vi "Find tab index.vi"(8 "error in (no error)":errorcluster, 11 "Save Image in":refnum<class "Save Image.lvclass">) -> (0 "error out":errorcluster, 1 "column":i32, 2 "row":i32, 3 "Save Image out":refnum<class "Save Image.lvclass">)   [LabVIEW 2018, in "Save Image.lvclass"]
uses:
  Save Image.lvclass
  Save Image.lvclass/Save Image.ctl
  Simulated_Header/Simulated_Header.lvclass
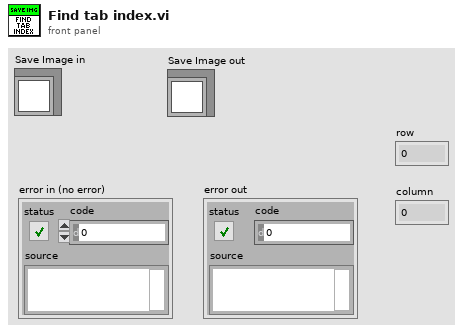
[diagram p1: front panel]
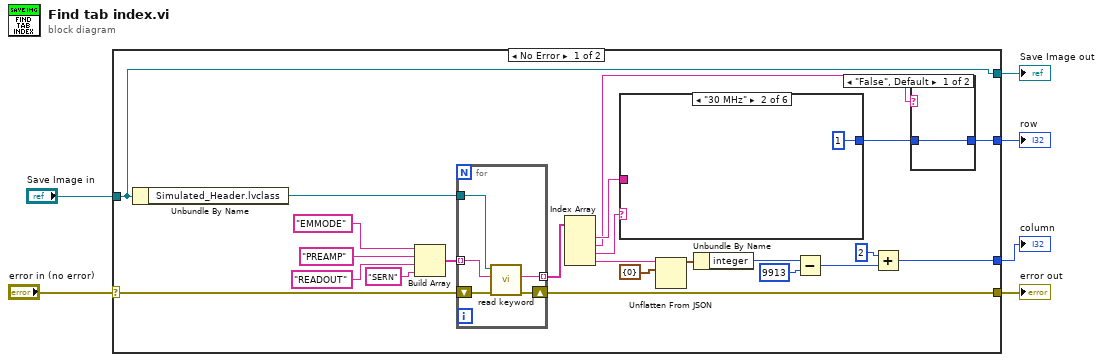
[diagram p0: block diagram]
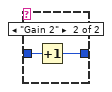
[diagram p2: hidden frame]
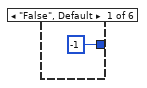
[diagram p3: hidden frame]
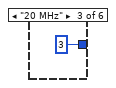
[diagram p4: hidden frame]
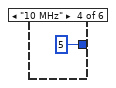
[diagram p5: hidden frame]
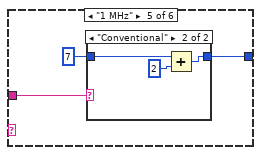
[diagram p6: hidden frame]
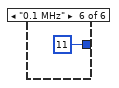
[diagram p8: hidden frame]
diagram:
  n1 = case shown="No Error" "error in (no error)" {
    selector: "error in (no error)" -> [w8 w50]
    tunnel: [w7 w51] -> w6
    tunnel: [w20 w50] -> w3
    tunnel: "Save Image in" -> [w7 w51]
    tunnel: [w11 _] -> w2
    tunnel: [w10 _] -> w1
    frame No Error {
      n2 = Unbundle By Name(w7) -> ("Simulated_Header.lvclass"=w9:refnum<class "Simulated_Header.lvclass">)
      n3 = Build Array("EMMODE", "PREAMP", "READOUT", "SERN") -> (w21:string[])
      n4 = for {
        tunnel: w9 -> [w34]
        tunnel: w21 -> [w33] mode=indexing
        tunnel: [w32] -> w19 mode=indexing
        shift-right: [w30] -> w20
        shift-left: w8 -> [w31]
        n5 = call "read keyword.vi"("error in (no error)"=w31, "keyword"=w33, "Simulated_Header in"=w34) -> ("error out"=w30:errorcluster, "value"=w32:string)  [unwired: 6 in, 1 out]
      }
      n6 = Index Array(array=w19) -> (element #1=w17:string, element #2=w16:string, element #3=w18:string, element #4=w15:string)  [unwired: 4 in]
      n7 = case shown="\"30 MHz\"" w18 {
        tunnel: [-1 ("index (row)") 1 ("index (row)") 3 ("index (row)") 5 ("index (row)") w42 11 ("index (row)")] -> w27
        tunnel: w17 -> [_ _ _ _ w44 _]
        frame "False", Default {
        }
        frame "30 MHz" {
        }
        frame "20 MHz" {
        }
        frame "10 MHz" {
        }
        frame "1 MHz" {
          n8 = case shown="\"Conventional\"" w44 {
            tunnel: 7 ("index (row)") -> [w45 w48]
            tunnel: [w45 w47] -> w42
            frame "False", Default {
            }
            frame "Conventional" {
              n9 = Add(x=w48, y=2 ("index (row)")) -> (x+y=w47:i32)
            }
          }
        }
        frame "0.1 MHz" {
        }
      }
      n10 = Unflatten From JSON(JSON string=w15, type and defaults=cluster{"integer":i32} {"integer"=0}) -> (value=w13:cluster{"integer":i32})  [unwired: 5 in, 1 out]
      n11 = Unbundle By Name(w13) -> ("integer"=w12:i32)
      n12 = Subtract(x=w12, y=9913 ("index (row)")) -> (x-y=w29:i32)
      n13 = Add(x=2 ("index (row)"), y=w29) -> (x+y=w10:i32)
      n14 = case shown="\"False\", Default" w16 {
        tunnel: w27 -> [w35 w37]
        tunnel: [w35 w36] -> w11
        frame "False", Default {
        }
        frame "Gain 2" {
          n15 = Increment(x=w37) -> (x+1=w36:i32)
        }
      }
    }
    frame Error {
    }
  }
  "Save Image out" <- w6
  "error out" <- w3
  "row" <- w2
  "column" <- w1
